vi "PiezoInit.vi"(0 "reference":refnum<k7>, 1 "HWSerialNum":i32=91897094, 3 "error in (no error)":errorcluster) -> (7 "reference out":refnum<k7>, 10 "error out":errorcluster)   [LabVIEW 2018]
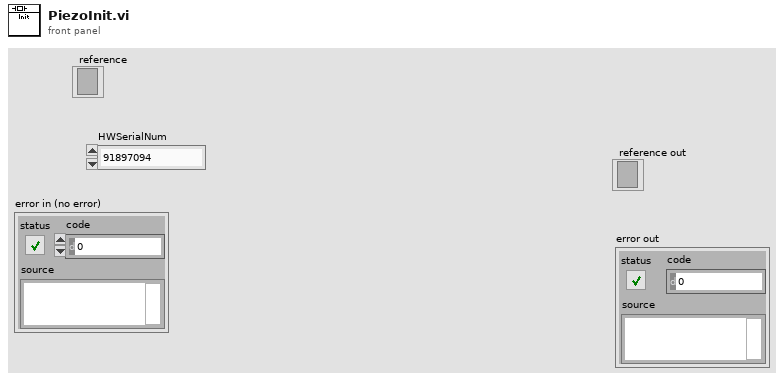
[diagram p1: front panel]
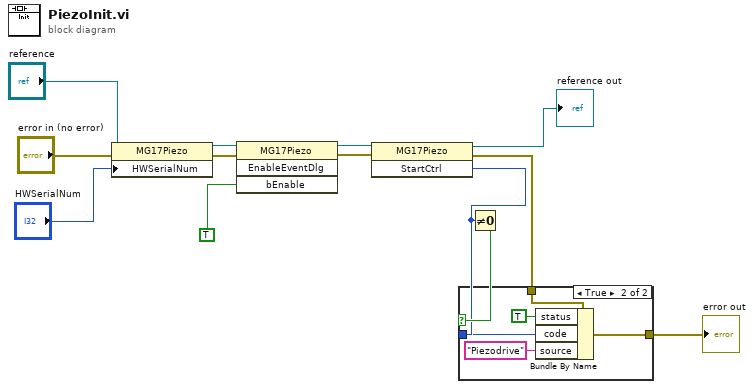
[diagram p0: block diagram]
diagram:
  n1 = property class="MG17Piezo"(reference="reference", error in="error in (no error)", "HWSerialNum"="HWSerialNum") -> (reference out=w5:refnum<k7>, error out=w4:errorcluster)
  n2 = invoke class="MG17Piezo" method="EnableEventDlg"(reference=w5, error in=w4, "bEnable"=TRUE) -> (reference out=w3:refnum<k7>, error out=w2:errorcluster)  [unwired: 1 in, 2 out]
  n3 = invoke class="MG17Piezo" method="StartCtrl"(reference=w3, error in=w2) -> (reference out=→"reference out":refnum<k7>, error out=w10:errorcluster, "StartCtrl"=w9:i32)  [unwired: 1 in]
  n4 = Not Equal To 0?(x=w9) -> (x != 0?=w11:bool)
  n5 = case shown="True" w11 {
    tunnel: w10 -> [w14 w19]
    tunnel: w9 -> [_ w17]
    tunnel: [w14 w15] -> w7
    frame False {
    }
    frame True {
      n6 = Bundle By Name(cluster=w19, "status"=TRUE, "code"=w17, "source"="Piezodrive") -> (w15:errorcluster)
    }
  }
  "error out" <- w7
